vi "Variant To Registry.vi"(4 "Registry Variant Accessor in":refnum<class "CConfig Variant Accessor.lvclass">, 6 "Variant":variant, 8 "error in (no error)":errorcluster, 9 "Create keys? [T]":bool=TRUE, 10 "Create sections? [T]":bool=TRUE, 11 "Carya Config in":refnum<class "Carya Config.lvclass">) -> (0 "error out":errorcluster, 1 "Created key?":bool, 2 "Created session?":bool, 3 "Carya Config out":refnum<class "Carya Config.lvclass">)   [LabVIEW 2013, in "Carya Config.lvclass"]
doc: "Copyright 2018, Carya Automatisering, Wiebe Walstra."
uses:
  Carya Config.lvclass
  CConfig Variant Accessor/CConfig Variant Accessor.lvclass
  CConfig Variant Accessor/CConfig Variant Accessor.lvclass/CConfig Variant Accessor.ctl
  <vilib>/Utility/error.llb/Error Cluster From Error Code.vi
  <vilib>/ErrorRing/Error Ring.xnode
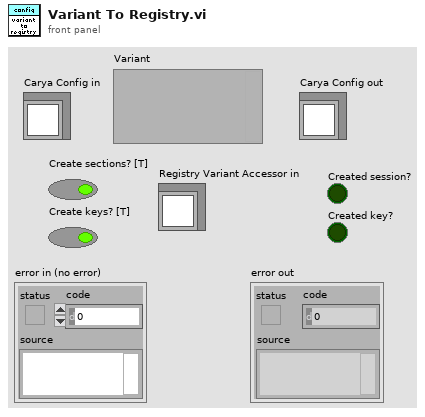
[diagram p1: front panel]
types:
  T1 = typedef "VariantType.lvlib/Type.ctl" = enum8{"Invalid Type", "Void", "I8", "I16", "I32", "I64", "U8", "U16", "U32", "U64", "Single Float", "Double Float", "Extended Float", "Single Complex", "Double Complex", "Extended Complex", "Enum U8", "Enum U16", "Enum U32", "Enum U64", "Single Float With Unit", "Double Float With Unit", "Extended Float With Unit", "Single Complex with Unit", "Double Complex with Unit", "Extended Complex with Unit", "Boolean", "String", "Path", "Picture", "Tag", "Array", "Cluster", "Variant", "LV Variant", "Waveform", "Timestamp", "Digital Waveform", "Digital Data", "ExpressData", "Refnum", "External Data", "VI", "Poly VI", "LabVIEW Class Instance", "Fixed Point"}
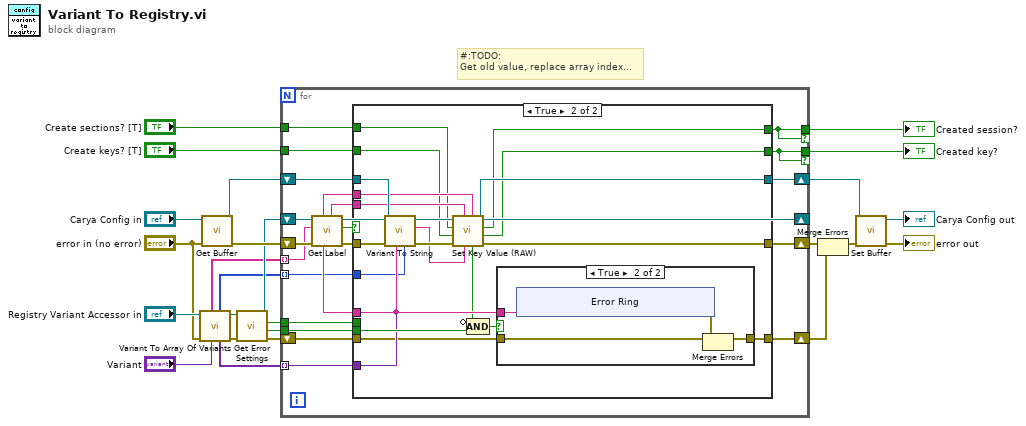
[diagram p0: block diagram]
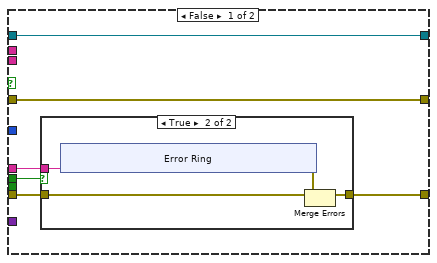
[diagram p2: hidden frame]
diagram:
  # "#:TODO:\nGet old value, replace array index..."
  n1 = call-dynamic "Variant To Array Of Variants.vi"("Variant"="Variant", "error in (no error)"="error in (no error)", "Registry Variant Accessor in"="Registry Variant Accessor in") -> ("error out"=w7:errorcluster, "Registry Variant Accessor out"=w20:refnum<class "CConfig Variant Accessor.lvclass">, "Variants"=w9:variant[], "Types"=w11:T1[], "Labels (RAW)"=w10:string[])  [unwired: 3 in, 1 out]
  n2 = call-dynamic "Get Buffer.vi"("error in (no error)"="error in (no error)", "Carya Config in"="Carya Config in") -> ("error out"=w13:errorcluster, "Config"=w2:refnum<class "Carya Config.lvclass">)  [unwired: 8 in]
  n3 = call "Get Error Settings.vi"("error in (no error)"=w7, "CConfig Variant Accessor in"=w20) -> ("error out"=w6:errorcluster, "Key not found error"=w18:bool, "Wrong label error"=w19:bool, "CConfig Variant Accessor out"=w12:refnum<class "CConfig Variant Accessor.lvclass">)  [unwired: 6 in]
  n4 = for {
    tunnel: w19 -> [w47]
    tunnel: w18 -> [w46]
    tunnel: "Create sections? [T]" -> [w44]
    tunnel: "Create keys? [T]" -> [w43]
    tunnel: [w39] -> w15 if=w39
    tunnel: [w40] -> w14 if=w40
    tunnel: w11 -> [w36] mode=indexing
    tunnel: w10 -> [w35] mode=indexing
    tunnel: w9 -> [w34] mode=indexing
    shift-right: [w33] -> w1
    shift-left: w2 -> [w45]
    shift-right: [w31] -> w4
    shift-left: w6 -> [w32]
    shift-right: [w30] -> w5
    shift-left: w13 -> [w38]
    shift-right: [w26] -> _
    shift-left: w12 -> [w37]
    n5 = call-dynamic "Get Label.vi"("error in (no error)"=w38, "Label"=w35, "Registry Variant Accessor in"=w37) -> ("error out"=w41:errorcluster, "Valid?"=w27:bool, "Registry Variant Accessor out"=w26:refnum<class "CConfig Variant Accessor.lvclass">, "Section out"=w29:string, "Complete label"=w42:string, "Key out"=w28:string)  [unwired: 3 in]
    n6 = case shown="True" w27 {
      tunnel: [w52 w80] -> w33
      tunnel: w41 -> [w48 w86]
      tunnel: w29 -> [_ w83]
      tunnel: w28 -> [_ w82]
      tunnel: w45 -> [w52 w85]
      tunnel: w42 -> [w53 w76]
      tunnel: [_ w78] -> w39
      tunnel: [_ w77] -> w40
      tunnel: w47 -> [w51 _]
      tunnel: w46 -> [_ w74]
      tunnel: w44 -> [_ w72]
      tunnel: w43 -> [_ w71]
      tunnel: w36 -> [_ w70]
      tunnel: w34 -> [_ w69]
      tunnel: w32 -> [w50 w68]
      tunnel: [w49 w67] -> w31
      tunnel: [w48 w66] -> w30
      frame False {
        n7 = case shown="True" w51 {
          tunnel: w53 -> [_ w57]
          tunnel: w50 -> [w54 w56]
          tunnel: [w54 w55] -> w49
          frame False {
          }
          frame True {
            n8 = xnode "Error Ring"("parameter 0"=w57) -> ("error out"=w58:errorcluster)
            n9 = Merge Errors(w56, w58) -> (w55:errorcluster)
          }
        }
      }
      frame True {
        n10 = call-dynamic "Variant To String.vi"("Type Enum [auto]"=w70, "Variant Type\\default"=w69, "Name (error)"=w76, "error in (no error)"=w86, "Registry Object"=w85) -> ("error out"=w84:errorcluster, "String"=w79:string, "Registry Object"=w81:refnum<class "Carya Config.lvclass">)  [unwired: 4 in]
        n11 = call-dynamic "Set Key Value (RAW).vi"("Key name"=w82, "Key value"=w79, "Section name"=w83, "error in (no error)"=w84, "Create key? [T]"=w71, "Create section? [T]"=w72, "Carya Config in"=w81) -> ("error out"=w66:errorcluster, "Created key?"=w77:bool, "Created session?"=w78:bool, "Carya Config out"=w80:refnum<class "Carya Config.lvclass">, "Value written?"=w75:bool)
        n12 = Compound Arithmetic op=AND(invert w75, w74) -> (w73:bool)
        n13 = case shown="True" w73 {
          tunnel: w76 -> [_ w90]
          tunnel: w68 -> [w87 w89]
          tunnel: [w87 w88] -> w67
          frame False {
          }
          frame True {
            n14 = xnode "Error Ring"("parameter 0"=w90) -> ("error out"=w91:errorcluster)
            n15 = Merge Errors(w89, w91) -> (w88:errorcluster)
          }
        }
      }
    }
  }
  "Created key?" <- w14
  "Created session?" <- w15
  n16 = Merge Errors(w5, w4) -> (w3:errorcluster)
  n17 = call-dynamic "Set Buffer.vi"("error in (no error)"=w3, "Carya Config"=w1) -> ("error out"=→"error out":errorcluster, "Carya Config out"=→"Carya Config out":refnum<class "Carya Config.lvclass">)  [unwired: 8 in]
